vi "tag select name change.vi"(8 "error in":errorcluster, 9 "new name":string, 10 "old name":string, 11 "object ref in":T1) -> (0 "error out":errorcluster, 2 "changed":bool, 3 "object ref out":T1)   [LabVIEW 2013]
uses:
  module/configuration/tag select module configuration.lvclass
  <vilib>/NI/Tag Bus Data Framework/Configuration Editor/Classes/Engine Parent/Engine Parent Editor Node.lvclass
  <vilib>/NI/Configuration Framework/serializable configuration/NISE_CEF_serializable configuration.lvclass
  <vilib>/NI/Module Execution Interface/Engine Configuration/engine configuration.lvclass
  <vilib>/NI/Tag Bus Data Framework/Configuration Editor/Classes/Module editor node/module editor node.lvclass
  <vilib>/NI/DCAF Table API/Table Manager/object ref.ctl
  <vilib>/NI/DCAF Table API/Table Manager/Table Manager.lvclass
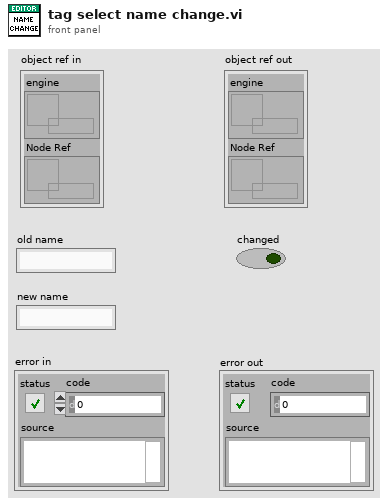
[diagram p1: front panel]
types:
  T1 = typedef "Table Manager.lvlib/Table Manager.lvclass/object ref.ctl" = cluster{"engine":refnum<data-value>, "Node Ref":refnum<data-value>}
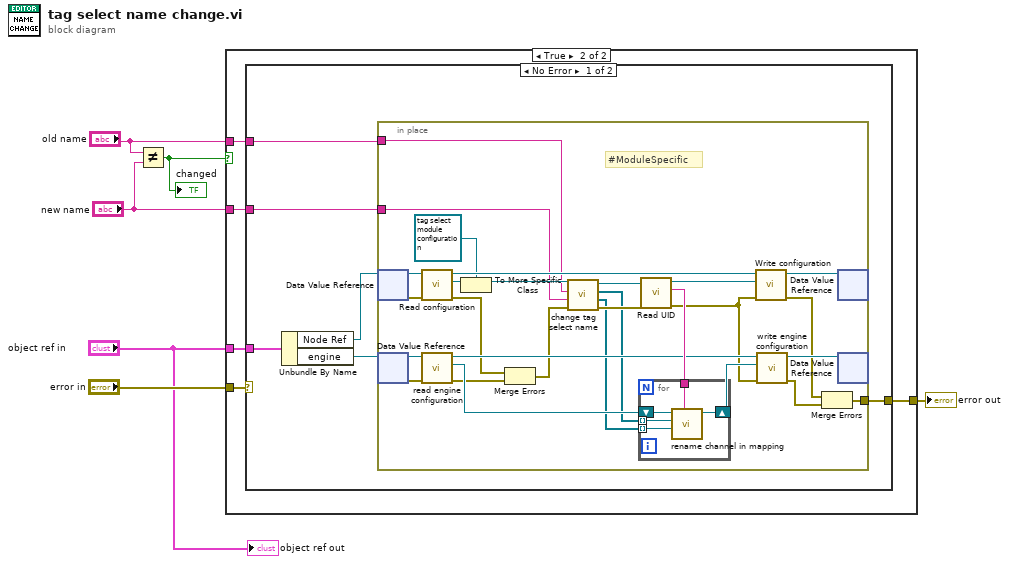
[diagram p0: block diagram]
diagram:
  n1 = Not Equal?(x="old name", y="new name") -> (x != y?=w3:bool)
  "changed" <- w3
  n2 = case shown="True" w3 {
    tunnel: "object ref in" -> [_ w12]
    tunnel: [w7 w11] -> w6
    tunnel: "error in" -> [w7 w10]
    tunnel: "old name" -> [_ w9]
    tunnel: "new name" -> [_ w8]
    frame False {
    }
    frame True {
      n3 = case shown="No Error" w10 {
        selector: w10 -> [_ w52]
        tunnel: w12 -> [w16 _]
        tunnel: [w15 w52] -> w11
        tunnel: w9 -> [w14 _]
        tunnel: w8 -> [w13 _]
        frame No Error {
          n4 = Unbundle By Name(w16) -> ("Node Ref"=w17:refnum<data-value>, "engine"=w18:refnum<data-value>)
          n5 = in-place {
            in-place-border: [w33] -> w15
            in-place-border: w14 -> [w22]
            in-place-border: w13 -> [w21]
            # "#ModuleSpecific"
            n6 = in-place-dvr #1(w17) -> (w27:refnum<class "module editor node.lvclass">, w32:errorcluster)
            n7 = in-place-dvr #2(w18) -> (w45:refnum<class "Engine Parent Editor Node.lvclass">, w46:errorcluster)
            n8 = call-dynamic "Read configuration.vi"("error in"=w32, "NISE_CEF_serializable node in"=w27) -> ("error out"=w31:errorcluster, "configuration"=w28:refnum<class "NISE_CEF_serializable configuration.lvclass">, "NISE_CEF_serializable node out"=w37:refnum<class "module editor node.lvclass">)  [unwired: 7 in]
            n9 = call <vilib>:"read engine configuration.vi"("error in"=w46, "Engine Parent Editor Node in"=w45) -> ("error out"=w40:errorcluster, "engine configuration"=w41:refnum<class "engine configuration.lvclass">, "Engine Parent Editor Node out"=w38:refnum<class "Engine Parent Editor Node.lvclass">)  [unwired: 7 in]
            n10 = To More Specific Class(target class=refnum<class "tag select module configuration.lvclass"> refnum ("tag select  module configuration in"), reference=w28) -> (specific class reference=w26:refnum<class "tag select module configuration.lvclass">)  [unwired: 1 in, 1 out]
            n11 = Merge Errors(w31, w40) -> (w25:errorcluster)
            n12 = call "change tag select name.vi"("error in"=w25, "new name"=w21, "old name"=w22, "tag select module configuration in"=w26) -> ("error out"=w24:errorcluster, "new channels"=w19:refnum<class "TBM channel.lvclass">[], "old channels"=w20:refnum<class "TBM channel.lvclass">[], "tag select module configuration out"=w23:refnum<class "tag select module configuration.lvclass">)  [unwired: 4 in]
            n13 = call <vilib>:"Read UID.vi"("error in"=w24, "configuration in"=w23) -> ("error out"=w30:errorcluster, "instance id"=w42:string, "configuration out"=w36:refnum<class "tag select module configuration.lvclass">)  [unwired: 7 in]
            n14 = for {
              shift-right: [w50] -> w39
              shift-left: w41 -> [w51]
              tunnel: w42 -> [w49]
              tunnel: w20 -> [w48] mode=indexing
              tunnel: w19 -> [w47] mode=indexing
              n15 = call <vilib>:"rename channel in mapping.vi"("owner ID"=w49, "new channel"=w47, "old channel"=w48, "engine configuration in"=w51) -> ("engine configuration out"=w50:refnum<class "engine configuration.lvclass">)  [unwired: 6 in, 1 out]
            }
            n16 = call-dynamic "Write configuration.vi"("error in"=w30, "configuration"=w36, "NISE_CEF_serializable node in"=w37) -> ("error out"=w34:errorcluster, "NISE_CEF_serializable node out"=w43:refnum<class "module editor node.lvclass">)  [unwired: 7 in]
            n17 = call <vilib>:"write engine configuration.vi"("error in"=w30, "engine configuration"=w39, "Engine Parent Editor Node in"=w38) -> ("error out"=w35:errorcluster, "Engine Parent Editor Node out"=w44:refnum<class "Engine Parent Editor Node.lvclass">)  [unwired: 7 in]
            n18 = Merge Errors(w34, w35) -> (w33:errorcluster)
            n19 = in-place-dvr #1(w43) -> ()  [unwired: 2 out]
            n20 = in-place-dvr #2(w44) -> ()  [unwired: 2 out]
          }
        }
        frame Error {
        }
      }
    }
  }
  "error out" <- w6
  "object ref out" <- "object ref in"
